vi "Sub_Build_Fixed_Header.vi"(6 "Remaining Length":u32, 8 "error in (no error)":errorcluster, 11 "MessageType":T1=enum."CONNECT") -> (0 "error out":errorcluster, 3 "Fixed Header":u8[](array[numeric]) format="%x")   [LabVIEW 2013, in "IOTFoundation.lvlib"]
uses:
  IOTFoundation.lvlib
  Controls/MessageType.ctl
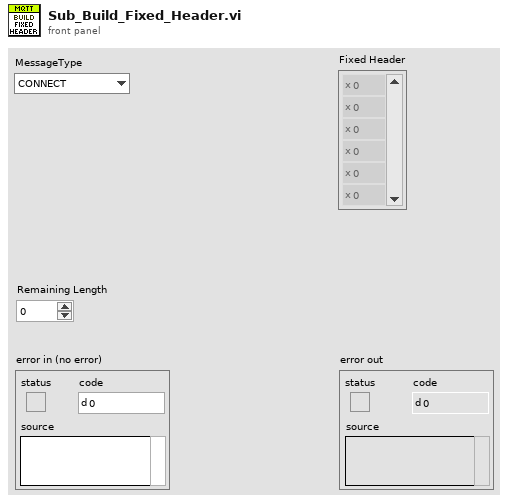
[diagram p1: front panel]
types:
  T1 = typedef "IOTFoundation.lvlib/MessageType.ctl" = enum32{"Reserved", "CONNECT", "CONNACK", "PUBLISH", "PUBACK", "PUBREC", "PUBREL", "PUBCOMP", "SUBSCRIBE", "SUBACK", "UNSUBSCRIBE", "UNSUBACK", "PINGREQ", "PINGRESP", "DISCONNECT", "Reserved2"}
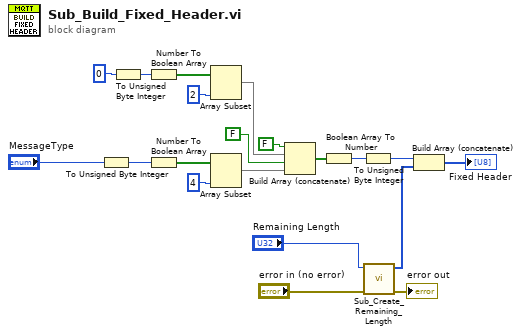
[diagram p0: block diagram]
diagram:
  n1 = To Unsigned Byte Integer(number="MessageType") -> (unsigned 8bit integer=w19:u8)
  n2 = To Unsigned Byte Integer(number=0) -> (unsigned 8bit integer=w18:u8)
  n3 = Number To Boolean Array(number=w18) -> (Boolean array=w15:bool[])
  n4 = Number To Boolean Array(number=w19) -> (Boolean array=w17:bool[])
  n5 = Array Subset(array=w15, length=2) -> (w5:bool[])  [unwired: 1 in]
  n6 = Array Subset(array=w17, length=4) -> (w4:bool[])  [unwired: 1 in]
  n7 = Build Array (concatenate)(FALSE, w5, FALSE, w4) -> (w13:bool[])
  n8 = Boolean Array To Number(Boolean array=w13) -> (number=w12:u32)
  n9 = To Unsigned Byte Integer(number=w12) -> (unsigned 8bit integer=w11:u8)
  n10 = call "Sub_Create_Remaining_Length.vi"("error in (no error)"="error in (no error)", "X"="Remaining Length") -> ("error out"=→"error out":errorcluster, "bytes"=w10:u8[])  [unwired: 8 in]
  n11 = Build Array (concatenate)(w11, w10) -> (→"Fixed Header":u8[])
